vi "Coherent comms (direct) L1.vi"(7 "Coherent laser commands L1":T4, 8 "error in (no error)":errorcluster, 10 "Commands \nand Queries":T1[](array[typedef]), 11 "Visa resource":T3) -> (0 "error out":errorcluster, 1 "Response":string[](array[string]), 2 "Resp Validated ?":bool[](array[boolean]), 3 "Data":string[](array[string]), 5 "VISA resource name out":refnum<visa-resource-name>)   [LabVIEW 2017]
uses:
  Type defs/Coherent comms control.ctl
  Serial Comms/Visa resource.ctl
  Type defs/Coherent commands direct mode.ctl
  Type defs/Commands List.ctl
  Serial Comms/Serial - Settings.ctl
panel:
  out "output cluster":cluster{bool, i32, bool, i32}
  out "return count":u32
  out "length":i32
  out "bytes read":u32
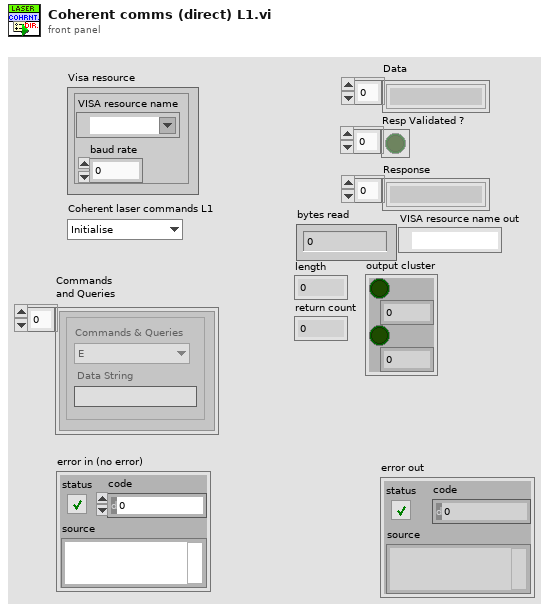
[diagram p1: front panel]
types:
  T1 = typedef "Coherent commands direct mode.ctl" = cluster{"Commands & Queries":T2, "Data String":string}
  T2 = typedef "Commands List.ctl" = enum16{"E", "B", "FL", "HM", "L", "LBOH", "LBOOPT", "LFP", "PROMPT", "SM", "S", "VW", "VWS", "HB", "HBR", "REQ", "ALIGN", "K", "F", "FH", "UF", "PHLDC", "PZTMC", "PZTXC", "PZTYC", "PHLDP", "PZTMP", "PZTXP", "PZTYP", "PTRK", "MDLK", "PP", "TS", "STPRPOS", "C", "D1C", "D2C", "BT", "D1T", "D2T", "VT", "LBOT", "ET", "D1ST", "D2ST", "VST", "LBOST", "EST", "D1TD", "D2TD", "VD", "LBOD", "ED", "D1HST", "D2HST", "LRS", "D1SS", "D2SS", "VSS", "LBOSS", "ESS", "D1H", "D2H", "HH", "D1V", "D2V", "SV", "MB", "PI", "BV", "AMDLK", "PZTS", "TMAX", "TMIN", "ALIGNP", "ALIGNW", "PZTXCM", "PZTXCP", "PZTXPM", "PZTXPP", "PZTYCM", "PZTYCP", "PZTYPM", "PZTYPP", "RH", "SN", "ST", "GDDCURVE", "GDD", "GDDCURVEN", "SETCURVEN", "SETCURVEPT", "SAVECURVE", "DELCURVE", "CURVEN", "CURVEPT", "CURVE", "COMP", "HMCOMP", "GDDMAX", "GDDMIN"}
  T3 = typedef "Visa resource.ctl" = cluster{"VISA resource name":refnum<visa-resource-name>, "baud rate":u32}
  T4 = typedef "Coherent comms control.ctl" = enum16{"Initialise", "Get Command", "Set Command", "Clear Buffer", "Close"}
  T5 = enum16{"Initialise", "Read Handle", "Command & Query", "Close"}
  T6 = typedef "Serial - Settings.ctl" = cluster{"VISA resource name ":refnum<visa-resource-name>, "baud rate":u32, "data bits":u16, "parity":enum16{"None", "Odd", "Even", "Mark", "Space"}, "stop bits":u16, "flow control":u16}
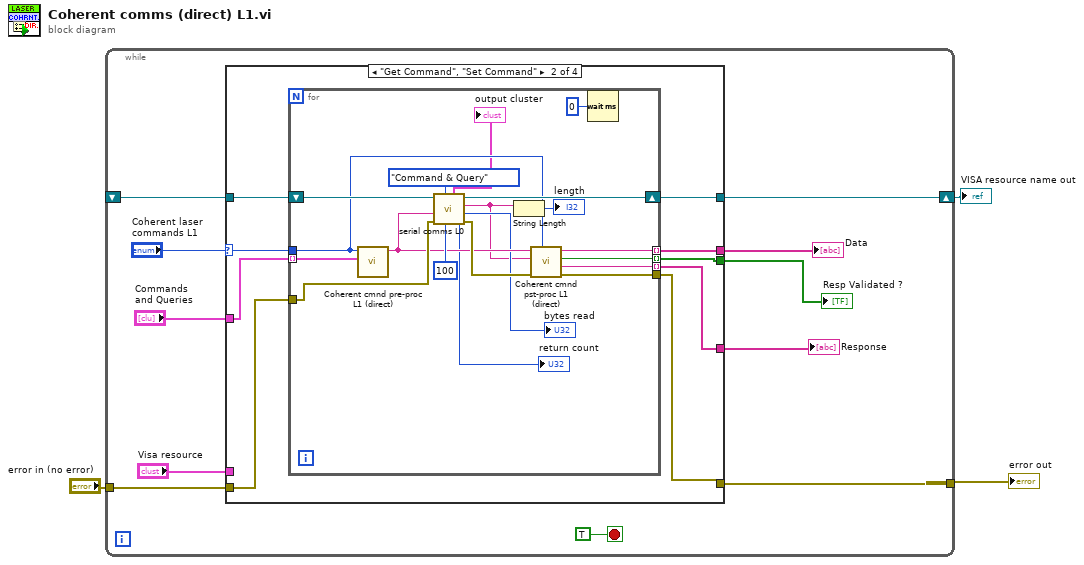
[diagram p0: block diagram]
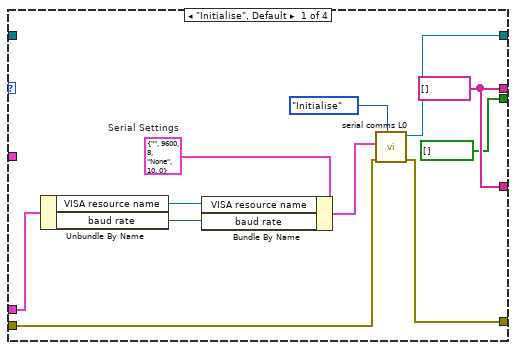
[diagram p2: hidden frame]
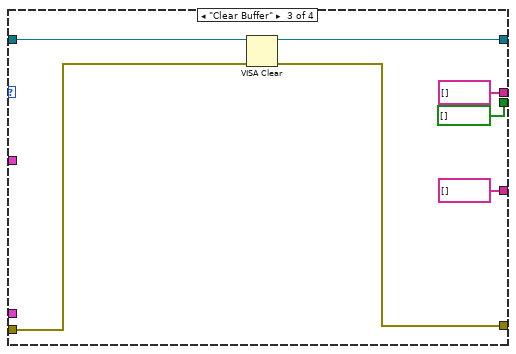
[diagram p3: hidden frame]
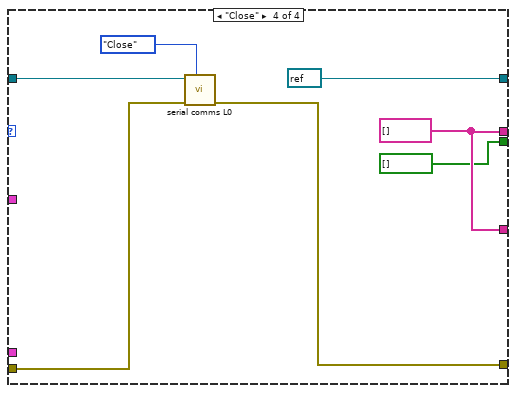
[diagram p4: hidden frame]
diagram:
  n1 = while {
    tunnel: "error in (no error)" -> [w13]
    tunnel: [w12] -> w2
    shift-right: [w9] -> w1
    shift-left: _ -> [w8]
    stop <- TRUE stop-if-true
    n2 = case shown="\"Get Command\", \"Set Command\"" "Coherent laser commands L1" {
      selector: "Coherent laser commands L1" -> [_ w30 _ _]
      tunnel: w13 -> [w23 w33 w60 w65]
      tunnel: [w22 w29 w59 w64] -> w12
      tunnel: "Visa resource" -> [w21 _ _ _]
      tunnel: [w18 w32 w57 refnum<visa-resource-name> refnum ("VISA resource name out")] -> w9
      tunnel: w8 -> [_ w34 w58 w66]
      tunnel: "Commands \nand Queries" -> [_ w31 _ _]
      tunnel: [w16 w28 string[] [] w62] -> w6
      tunnel: [w16 w27 string[] [] w62] -> w5
      tunnel: [bool[] [] w26 bool[] [] bool[] []] -> w4
      frame "Initialise", Default {
        w16 = string[] []
        w25 = T6 {"VISA resource name "="", "baud rate"=9600, "data bits"=8, "parity"=enum."None", "stop bits"=10, "flow control"=0}  # Serial Settings
        n3 = Unbundle By Name(w21) -> ("VISA resource name"=w20:refnum<visa-resource-name>, "baud rate"=w19:u32)
        n4 = Bundle By Name(cluster=w25, "VISA resource name"=w20, "baud rate"=w19) -> (w24:T6)
        n5 = call "serial comms L0.vi"("Comms Control"=T5."Initialise", "error IN"=w23, "Serial Settings"=w24) -> ("Error OUT"=w22:errorcluster, "VISA resource name out"=w18:refnum<visa-resource-name>)  [unwired: 3 in, 4 out]
      }
      frame "Get Command", "Set Command" {
        n6 = for {
          tunnel: w33 -> [w52]
          shift-right: [w51] -> w32
          shift-left: w34 -> [w53]
          tunnel: w31 -> [w50] mode=indexing
          tunnel: w30 -> [w49]
          tunnel: [w48] -> w28 mode=indexing
          tunnel: [w47] -> w26 mode=indexing
          tunnel: [w46] -> w27 mode=indexing
          tunnel: [w45] -> w29
          n7 = call "Coherent cmnd pre-proc L1 (direct).vi"("Coherent Commands"=w50, "Coherent laser commands L1"=w49) -> ("concatenated string"=w40:string)  [unwired: 9 in]
          n8 = call "serial comms L0.vi"("delay before read (ms)"=u32 100, "Comms Control"=T5."Command & Query", "error IN"=w52, "Command String"=w40, "VISA resource name"=w53) -> ("Error OUT"=w41:errorcluster, "bytes read"=→"bytes read":u32, "Response"=w38:string, "VISA resource name out"=w51:refnum<visa-resource-name>, "return count"=→"return count":u32, "output cluster"=→"output cluster":cluster{bool, i32, bool, i32})  [unwired: 1 in]
          n9 = String Length(string=w38) -> (length=→"length":i32)
          n10 = call "Coherent cmnd pst-proc L1 (direct).vi"("Coherent laser commands L1"=w49, "error in (no error)"=w41, "Response String"=w38, "Command String"=w40) -> ("error out"=w45:errorcluster, "Response String"=w46:string, "Response Validated ?"=w47:bool, "trimmed string"=w48:string)  [unwired: 3 in, 1 out]
          n11 = Wait (ms)(milliseconds to wait=u32 0) -> ()  [unwired: 1 out]
        }
      }
      frame "Clear Buffer" {
        n12 = VISA Clear(VISA resource name=w58, error in (no error)=w60) -> (VISA resource name out=w57:refnum<visa-resource-name>, error out=w59:errorcluster)
      }
      frame "Close" {
        w62 = string[] []
        n13 = call "serial comms L0.vi"("Comms Control"=T5."Close", "error IN"=w65, "VISA resource name"=w66) -> ("Error OUT"=w64:errorcluster)  [unwired: 3 in, 5 out]
      }
    }
    "Data" <- w6
    "Response" <- w5
    "Resp Validated ?" <- w4
  }
  "error out" <- w2
  "VISA resource name out" <- w1
